vi "Commanded axes connected.vi"(0 "System no.":i32=1 min=1 max=4 step=1, 2 "Commanded axes":string[](array[string]), 5 "error in":errorcluster) -> (14 "Controller error":bool, 19 "error out":errorcluster)   [LabVIEW 2026]
doc: "This VI checks if Commanded axes are a subset of all connected axes (read from Global2 (Array).vi) and returns Controller error TRUE if this is not the case. Connected axes are defined by Define connected axes.vi which is called by PI_GCS2_Configuration_Setup.vi automatically. White space strings in Commanded axes are ignored."
panel:
  out "Conn. Axes":string[](array[string])
  # "This VI checks if commanded axes are a subset of all connected axes and returns \"Controller error\" TRUE if this is not the case. Connected axes are defined by Define connected axes.vi, which is called by \"XXX_Configuration_Setup.vi\" automatically. White space strings in \"Commanded axes\" are ignored."
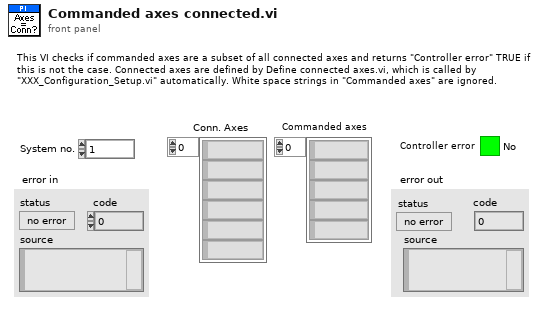
[diagram p1: front panel]
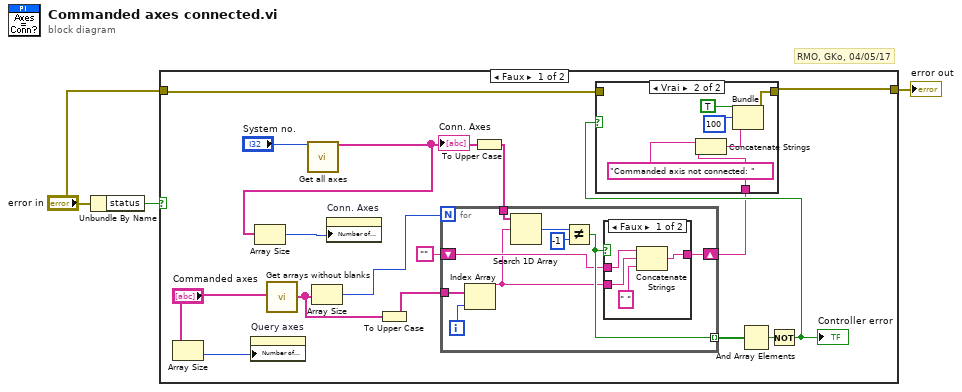
[diagram p0: block diagram]
diagram:
  # "RMO, GKo, 04/05/17"
  n1 = Unbundle By Name("error in") -> ("status"=w2:bool)
  n2 = case shown="Faux" w2 {
    tunnel: [w16 w41] -> w1
    tunnel: "error in" -> [w14 w41]
    frame False {
      n3 = Array Size(array="Commanded axes") -> (size(s)=w12:i32)
      n4 = property on="Query axes" class="Tabl (strict)"("Number of Rows"=w12) -> ()  [unwired: 2 in, 2 out]
      n5 = call "Get arrays without blanks.vi"("String array in"="Commanded axes") -> ("String array out"=w8:string[])  [unwired: 2 in, 16 out]
      n6 = call "Get all axes.vi"("System no."="System no.") -> ("Conn. Axes"=w6:string[])  [unwired: 18 out]
      "Conn. Axes" <- w6
      n7 = Array Size(array=w6) -> (size(s)=w13:i32)
      n8 = Array Size(array=w8) -> (size(s)=w7:i32)
      n9 = property on="Conn. Axes" class="Tabl (strict)"("Number of Rows"=w13) -> ()  [unwired: 2 in, 2 out]
      n10 = To Upper Case(1:w8) -> (0:w17:string[])
      n11 = To Upper Case(1:w6) -> (0:w10:string[])
      n12 = for {
        N: w7 -> [_]
        tunnel: w17 -> [w35]
        tunnel: [w32] -> w19 mode=indexing
        shift-right: [w30] -> w4
        shift-left: "" -> [w31]
        tunnel: w10 -> [w28]
        i -> [w34]
        n13 = Index Array(array=w35, index=w34) -> (element=w27:string)
        n14 = Search 1D Array(1D array=w28, element=w27) -> (index of element=w29:i32)  [unwired: 1 out]
        n15 = Not Equal?(x=w29, y=-1) -> (x != y?=w32:bool)
        n16 = case shown="Faux" w32 {
          tunnel: w31 -> [w38 w40]
          tunnel: [w37 w40] -> w30
          tunnel: w27 -> [w39 _]
          frame False {
            n17 = Concatenate Strings(w38, w39, " ") -> (w37:string)
          }
          frame True {
          }
        }
      }
      n18 = And Array Elements(Boolean array=w19) -> (logical AND=w18:bool)
      n19 = Not(x=w18) -> (.not. x?=w15:bool)
      "Controller error" <- w15
      n20 = case shown="Vrai" w15 {
        tunnel: [w20 w22] -> w16
        tunnel: w14 -> [w20 _]
        tunnel: w4 -> [_ w21]
        frame False {
        }
        frame True {
          n21 = Concatenate Strings("Commanded axis not connected: " ("source"), w21) -> (w23:string)
          n22 = Bundle("status"=TRUE, "code"=100, w23) -> (w22:cluster{"status":bool, "code":i32, string})  [unwired: 1 out]
        }
      }
    }
    frame True {
    }
  }
  "error out" <- w1
